vi "NativeVsFormulaNode.vi"(0 "Input X":dbl, 5 "Stop":bool) -> (4 "Y (Formula Method)":dbl, 6 "Y (Native Method)":dbl, 8 "Formula Method Time":dbl, 10 "Native Method Time":dbl, 15 "Fastest Method":string)   [LabVIEW 2020]
panel:
  # "Finding the fastest Method in labview"
  # "Result in every method"
  # "Time taken in every method"
  # "Description:\n1. This Vi helps to find which is the faster in means of execution speed. \n2. This shows the differnce between formula node and labview native node. \n3. The input formula is given in Numeric. Then using both the formula and labview native nodes. They are processed and shown in the near output bars.\n4. The fastest method is shown in the fastest method indicator."
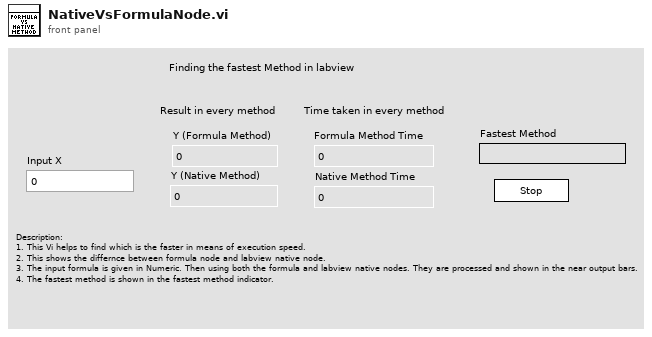
[diagram p1: front panel]
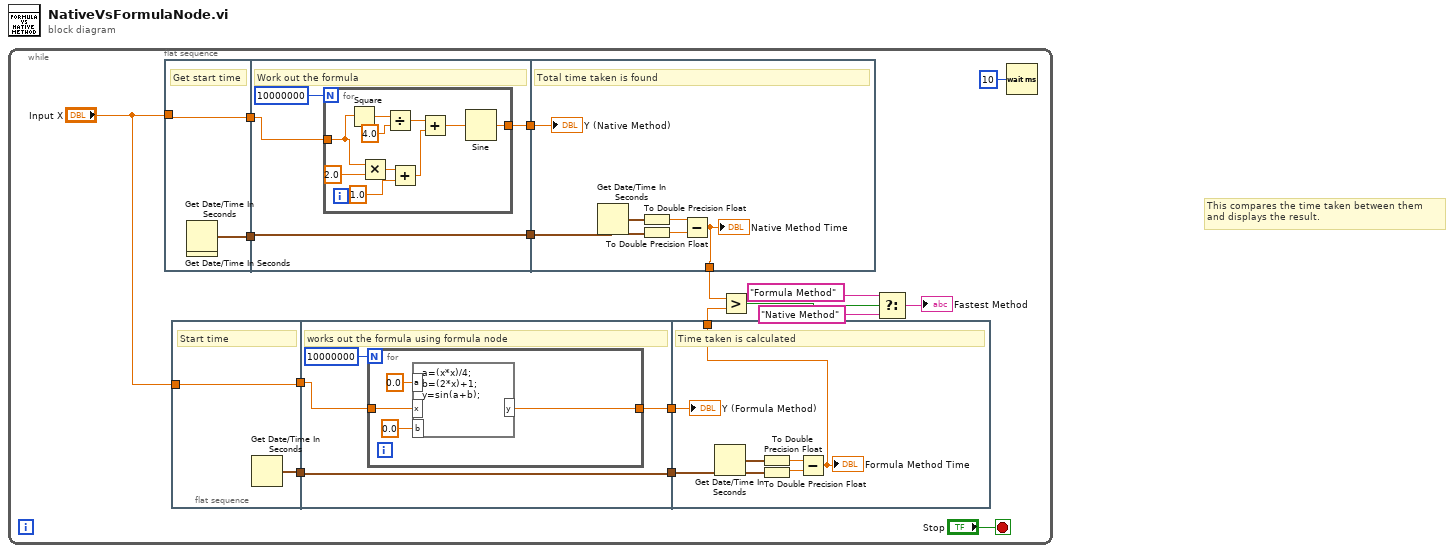
[diagram p0: block diagram]
diagram:
  # "This compares the time taken between them \nand displays the result."
  n1 = while {
    stop <- "Stop" stop-if-true
    n2 = flat-sequence {
      tunnel: [w34] -> w17
      tunnel: [w35] -> w16
      tunnel: "Input X" -> [w34]
      tunnel: [w39] -> w15
      tunnel: w17 -> [w38]
      tunnel: w16 -> [w37]
      tunnel: [w37] -> w14
      tunnel: w15 -> [w55]
      tunnel: w14 -> [w54]
      tunnel: [w50] -> w9
      frame #0 {
        # "Get start time"
        n3 = Get Date/Time In Seconds() -> (seconds since 1Jan1904=w35:timestamp)
        n4 = Get Date/Time In Seconds() -> ()  [unwired: 1 out]
      }
      frame #1 {
        # "Work out the formula"
        n5 = for {
          N: 10000000 -> [_]
          tunnel: w38 -> [w40]
          tunnel: [w41] -> w39
          n6 = Square(x=w40) -> (x^2=w49:dbl)
          n7 = Multiply(x=w40, y=2.0) -> (x*y=w46:dbl)
          n8 = Divide(x=w49, y=4.0) -> (x/y=w44:dbl)
          n9 = Add(x=w46, y=1.0) -> (x+y=w43:dbl)
          n10 = Add(x=w44, y=w43) -> (x+y=w42:dbl)
          n11 = Sine(x=w42) -> (sin(x)=w41:dbl)
        }
      }
      frame #2 {
        # "Total time taken is found"
        n12 = Get Date/Time In Seconds() -> (seconds since 1Jan1904=w52:timestamp)
        n13 = To Double Precision Float(number=w52) -> (double precision float=w51:dbl)
        n14 = To Double Precision Float(number=w54) -> (double precision float=w53:dbl)
        n15 = Subtract(x=w51, y=w53) -> (x-y=w50:dbl)
        "Native Method Time" <- w50
        "Y (Native Method)" <- w55
      }
    }
    n16 = flat-sequence {
      tunnel: [w19] -> w13
      tunnel: "Input X" -> [w18]
      tunnel: [w18] -> w12
      tunnel: w13 -> [w23]
      tunnel: [w23] -> w11
      tunnel: w12 -> [w21]
      tunnel: [w20] -> w3
      tunnel: w11 -> [w33]
      tunnel: w3 -> [w29]
      tunnel: [w28] -> w2
      frame #0 {
        # "Start time"
        n17 = Get Date/Time In Seconds() -> (seconds since 1Jan1904=w19:timestamp)
      }
      frame #1 {
        # "works out the formula using formula node"
        n18 = for {
          N: 10000000 -> [_]
          tunnel: w21 -> [w27]
          tunnel: [w24] -> w20
          n19 = formula code="a=(x*x)/4;\nb=(2*x)+1;\ny=sin(a+b);"("x"=w27, "a"=0.0 ("input variable"), "b"=0.0 ("input variable")) -> ("y"=w24:dbl)
        }
      }
      frame #2 {
        # "Time taken is calculated"
        n20 = Get Date/Time In Seconds() -> (seconds since 1Jan1904=w32:timestamp)
        n21 = To Double Precision Float(number=w32) -> (double precision float=w31:dbl)
        n22 = To Double Precision Float(number=w33) -> (double precision float=w30:dbl)
        n23 = Subtract(x=w31, y=w30) -> (x-y=w28:dbl)
        "Formula Method Time" <- w28
        "Y (Formula Method)" <- w29
      }
    }
    n24 = Greater?(x=w9, y=w2) -> (0:w8:bool)
    n25 = Select(t="Formula Method", s=w8, f="Native Method") -> (s? t:f=→"Fastest Method":string)
    n26 = Wait (ms)(milliseconds to wait=u32 10) -> ()  [unwired: 1 out]
  }
